vi "Request Data JSON.vi"(8 "error in (no error)":errorcluster, 11 "SetInputVolume in":refnum<class "SetInputVolume.lvclass">) -> (0 "error out":errorcluster, 2 "Request Data JSON":string, 3 "SetInputVolume out":refnum<class "SetInputVolume.lvclass">)   [LabVIEW 2020, in "obs-websocket.lvlib" / "SetInputVolume.lvclass"]
uses:
  SetInputVolume.lvclass
  SetInputVolume.lvclass/SetInputVolume.ctl
  9ff13f5e-cc8d-4f96-a5ad-0395e1bb4caa.vi
  <vilib>/JDP Science/JSONtext/Variant to JSON Text.vi
  <vilib>/JDP Science/JSONtext/LVClass Serializer/JSONtext LVClass Serializer.lvclass
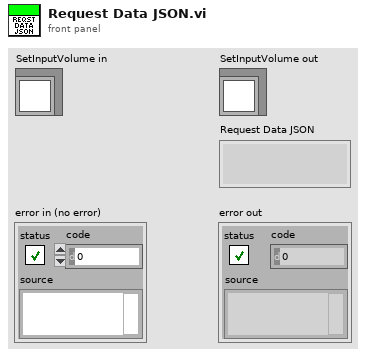
[diagram p1: front panel]
types:
  T1 = cluster{"inputVolumeMul":dbl, "inputName":string}
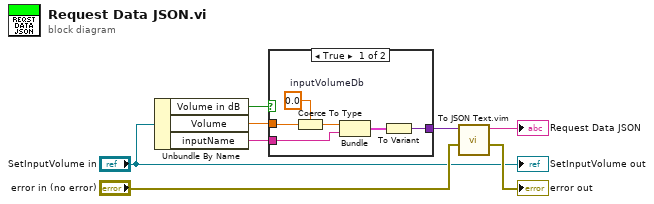
[diagram p0: block diagram]
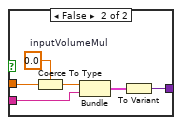
[diagram p2: hidden frame]
diagram:
  n1 = Unbundle By Name("SetInputVolume in") -> ("Volume in dB"=w3:bool, "Volume"=w4:dbl, "inputName"=w5:string)
  n2 = case shown="True" w3 {
    tunnel: w5 -> [w11 w17]
    tunnel: w4 -> [w14 w20]
    tunnel: [w9 w15] -> w2
    frame True {
      w13 = 0.0  # inputVolumeDb
      n3 = Coerce To Type(0:w14, 1:w13) -> (2:w12:dbl)
      n4 = Bundle("inputVolumeDb"=w12, "inputName"=w11) -> (w10:cluster{"inputVolumeDb":dbl, "inputName":string})  [unwired: 1 in]
      n5 = To Variant(anything=w10) -> (Variant=w9:variant)
    }
    frame False {
      w19 = 0.0  # inputVolumeMul
      n6 = Coerce To Type(0:w20, 1:w19) -> (2:w18:dbl)
      n7 = Bundle("inputVolumeMul"=w18, "inputName"=w17) -> (w16:T1)  [unwired: 1 in]
      n8 = To Variant(anything=w16) -> (Variant=w15:variant)
    }
  }
  n9 = call "To JSON Text.vim"("error in (no error)"="error in (no error)", "Anything"=w2) -> ("error out"=→"error out":errorcluster, "<JSON>"=→"Request Data JSON":string)  [unwired: 8 in]
  "SetInputVolume out" <- "SetInputVolume in"
